vi "ConvertToDtc.vi"(8 "error in":errorcluster {"code" format="%.0x"}, 11 "DataLineIn":string="59 02 09 95 72 47 21 01 08 95 75 00 08 47 22 95 76 54 09") -> (0 "error out":errorcluster {"code" format="%.0x"}, 1 "Lenght":i32, 2 "DtcLineOut":string, 3 "DtcItems":T1[](array[typedef]) {"Status Byte" format="%02x"})   [LabVIEW 2011, in "Konvolucio MUDS150628.lvlib"]
uses:
  <instrlib>/Konvolucio MUDS150628/Konvolucio MUDS150628.lvlib
  <instrlib>/Konvolucio MUDS150628/Types/DtcItemType.ctl
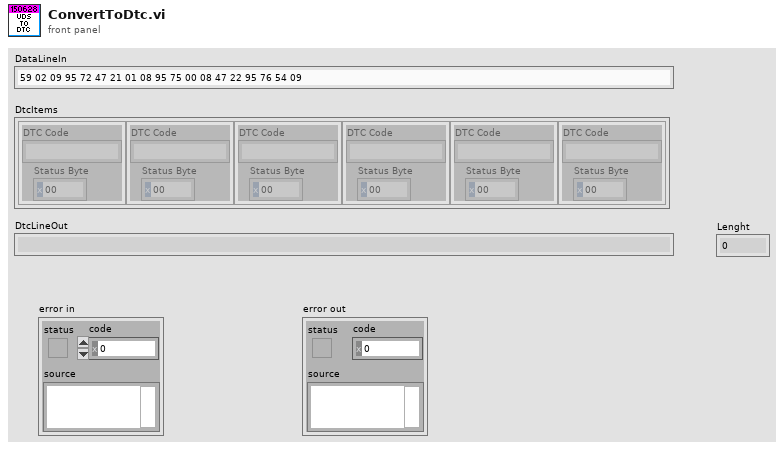
[diagram p1: front panel]
types:
  T1 = typedef "Konvolucio MUDS150628.lvlib/DtcItemType.ctl" = cluster{"DTC Code":string, "Status Byte":i32}
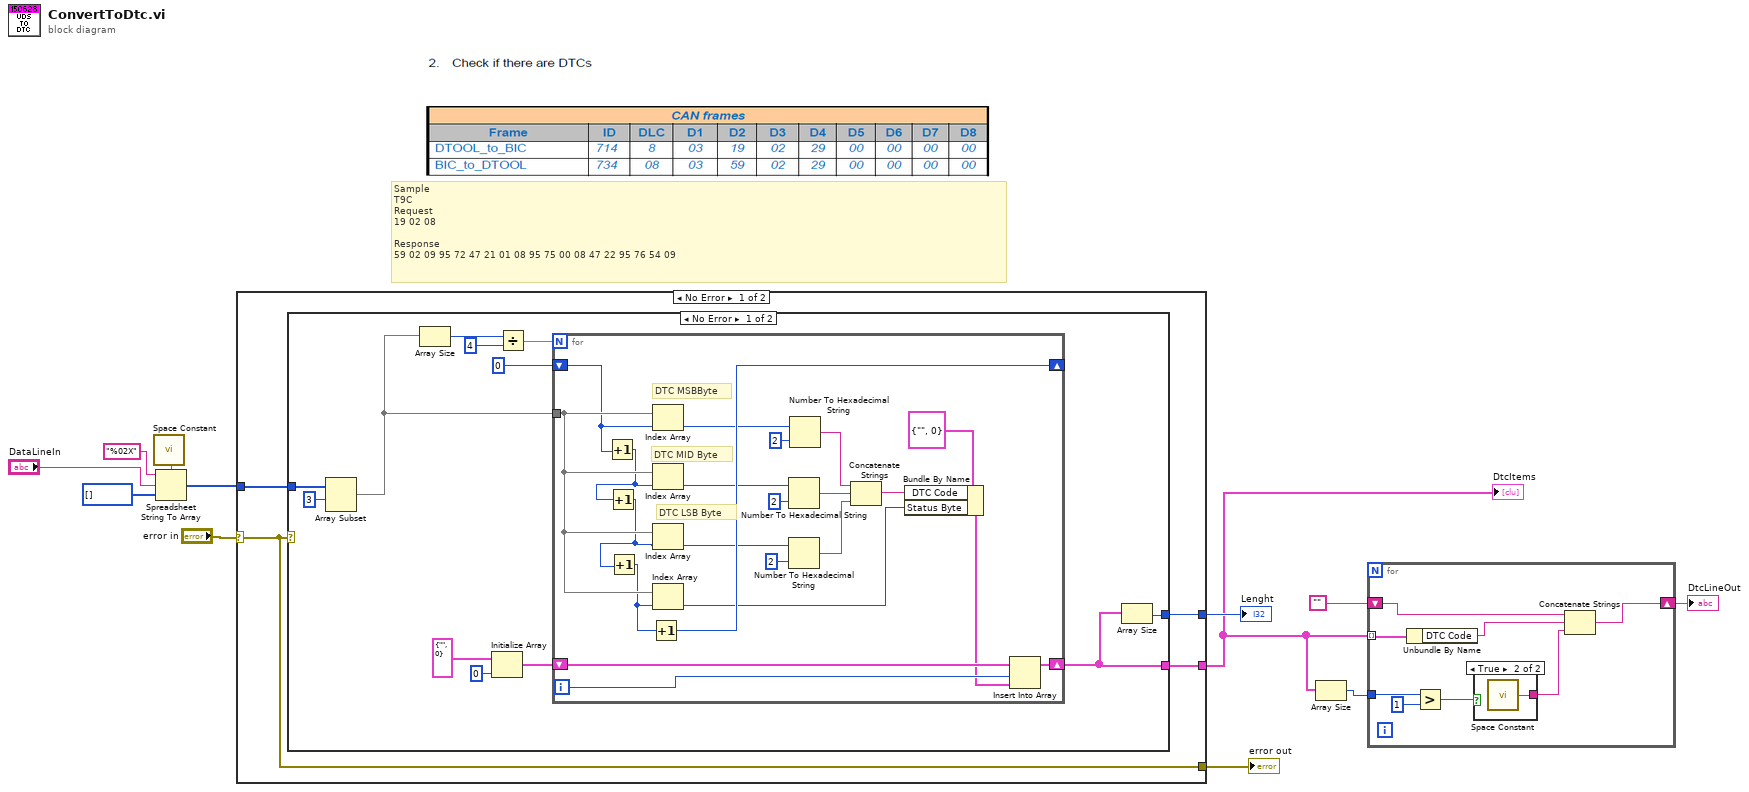
[diagram p0: block diagram]
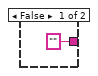
[diagram p2: hidden frame]
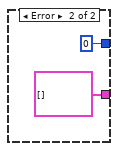
[diagram p3: hidden frame]
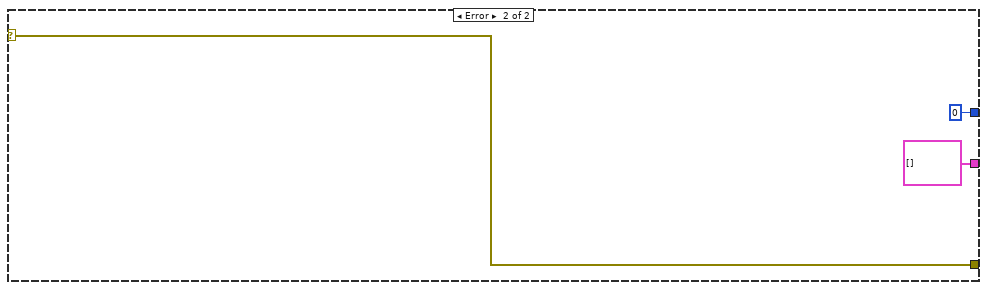
[diagram p4: hidden frame]
diagram:
  # "Sample\nT9C\nRequest  \n19 02 08\n\nResponse \n59 02 09 95 72 47 21 01 08 95 75 00 08 47 22 95 76 54 09"
  n1 = call <vilib>:"Space Constant.vi"() -> ("String"=w5:string)
  n2 = Spreadsheet String To Array(delimiter (Tab)=w5, format string="%02X", spreadsheet string="DataLineIn", array type (2D Dbl)=u8[] [] ("Response")) -> (array=w1:u8[])
  n3 = case shown="No Error" "error in" {
    selector: "error in" -> [w14 w53]
    tunnel: [w16 cluster{"DTC Code":string, "Status Byte":i32}[] []] -> w9
    tunnel: [w15 0] -> w11
    tunnel: [w14 w53] -> w12
    tunnel: w1 -> [w13 _]
    frame No Error {
      n4 = case shown="No Error" w14 {
        tunnel: w13 -> [w28 _]
        tunnel: [w19 cluster{"DTC Code":string, "Status Byte":i32}[] []] -> w16
        tunnel: [w18 0] -> w15
        frame No Error {
          n5 = Array Subset(array=w28, index=3) -> (w20:u8[])  [unwired: 1 in]
          n6 = Array Size(array=w20) -> (size(s)=w24:i32)
          n7 = Initialize Array(T1 {"DTC Code"="", "Status Byte"=0} ("DTC"), 0 ("dimension size")) -> (w21:T1[])
          n8 = Divide(x=w24, y=4) -> (x/y=w25:dbl)
          n9 = for {
            N: w25 -> [_]
            tunnel: w20 -> [w50]
            shift-right: [w45] -> _
            shift-left: 0 ("index") -> [w49]
            shift-right: [w43] -> w19
            shift-left: w21 -> [w44]
            i -> [w42]
            # "DTC LSB Byte"
            # "DTC MID Byte"
            # "DTC MSBByte"
            n10 = Increment(x=w49) -> (x+1=w48:i32)
            n11 = Increment(x=w48) -> (x+1=w47:i32)
            n12 = Increment(x=w47) -> (x+1=w46:i32)
            n13 = Increment(x=w46) -> (x+1=w45:i32)
            n14 = Index Array(array=w50, index=w49) -> (element=w40:u8)
            n15 = Index Array(array=w50, index=w48) -> (element=w38:u8)
            n16 = Index Array(array=w50, index=w47) -> (element=w36:u8)
            n17 = Index Array(array=w50, index=w46) -> (element=w31:u8)
            n18 = Number To Hexadecimal String(1:i16 2 ("width (-)"), 2:w38) -> (0:w33:string)
            n19 = Number To Hexadecimal String(1:i16 2 ("width (-)"), 2:w36) -> (0:w35:string)
            n20 = Number To Hexadecimal String(1:i16 2 ("width (-)"), 2:w40) -> (0:w34:string)
            n21 = Concatenate Strings(w34, w33, w35) -> (w32:string)
            n22 = Bundle By Name(cluster=T1 {"DTC Code"="", "Status Byte"=0} ("DTC"), "DTC Code"=w32, "Status Byte"=w31) -> (w30:T1)
            n23 = Insert Into Array(array=w44, index=w42, new element=w30) -> (w43:T1[])
          }
          n24 = Array Size(array=w19) -> (size(s)=w18:i32)
        }
        frame Error {
        }
      }
    }
    frame Error {
    }
  }
  "Lenght" <- w11
  "error out" <- w12
  "DtcItems" <- w9
  n25 = Array Size(array=w9) -> (size(s)=w8:i32)
  n26 = for {
    tunnel: w9 -> [w63] mode=indexing
    shift-right: [w57] -> w7
    shift-left: "" -> [w62]
    tunnel: w8 -> [w60]
    n27 = Unbundle By Name(w63) -> ("DTC Code"=w61:string)
    n28 = Greater?(x=w60, y=1) -> (0:w58:bool)
    n29 = case shown="True" w58 {
      tunnel: ["" w65] -> w56
      frame False {
      }
      frame True {
        n30 = call <vilib>:"Space Constant.vi"() -> ("String"=w65:string)
      }
    }
    n31 = Concatenate Strings(w62, w61, w56) -> (w57:string)
  }
  "DtcLineOut" <- w7
